vi "CR-导丝划痕检测1.vi"(8 "error in (no error)":errorcluster caption="错误输入（无错误）", 11 "名称或相对路径":string="Template Program") -> (0 "error in (no error) 2":errorcluster caption="错误输入（无错误）")   [LabVIEW 2017]
uses:
  Picture/SaveButtom.ctl
  Global System.vi
  <vilib>/Utility/xml.llb/Write to XML File(string).vi
panel:
  in  "获取图像":bool
  in  "ROI获取":bool
  in  "创建模板":bool
  in  "保存图像":bool
  out "添加的路径":path
  in  "刷新":bool
  in  "测试按钮":bool
  in  "保存按钮":bool
  in  "Main":enum32{"主参数", "模板匹配参数 ", "测试效果"}(tab)
  in  "导丝划痕检测1基础参数":T1={"IsNorImage"=TRUE, "Exposure Values"=100289, "ImagePath"=path "C:/Users/hedongpo/Desktop/514-hdp/Alignment Assemble System/Test Picture/B/3.bmp"} caption="参数界面" {"Exposure Values" scale=0.0..200000.0}
  in  "导丝划痕检测1参数":T3={"Rectangle"={"Left"=0, "Top"=0, "Right"=0, "Bottom"=0, "Rotation"=0.0}, "Algorithm "=2, "Parameters"={"Number of Matches Requested"=1, "Minimum Match Score"=800.0, "Angle Ranges"=[{"Start Angle"=-180.0, "End Angle"=180.0}]}, "Advanced Options "=[{"Item"=102, "Value"=10.0}, {"Item"=106, "Value"=300.0}, {"Item"=107, "Value"=0.0}, {"Item"=108, "Value"=6.0}, {"Item"=109, "Value"=1.0}, {"Item"=114, "Value"=25.0}, {"Item"=111, "Value"=20.0}, {"Item"=112, "Value"=10.0}, {"Item"=113, "Value"=20.0}, {"Item"=103, "Value"=1.0}, {"Item"=104, "Value"=20.0}, {"Item"=105, "Value"=0.0}, {"Item"=100, "Value"=5.0}], "模板路径"=path "", "Color Plane "=0} {"Color Plane" items=["Red", "Green", "Blue", "Hue", "Saturation", "Luminance", "Value", "Intensity"]; "Advanced Options"."Item" items=["LD Sampling - Minimum Constrast"=0, "LD Sampling - Enable Subpixel Accuracy"=1, "LD Sampling - Search Strategy"=2, "LD Sampling - Subpixel Iterations"=3, "LD Sampling - Subpixel Tolerance"=4, "LD Sampling - Initial Match List Length"=5, "LD Sampling - Match List Reduction Factor"=6, "LD Sampling - Initial Step Size"=7, "LD Sampling - Intermediate Angular Accuracy"=8, "-"=9, "Pyramid - Max Pyramid Level"=100, "Pyramid - Minimum Contrast"=102, "Pyramid - Enable Subpixel Accuracy"=103, "Pyramid - Subpixel Iterations"=104, "Pyramid - Subpixel Tolerance"=105, "Pyramid - Initial Match List Length"=106, "Pyramid - Match List Reduction Factor"=107, "Pyramid - Intermediate Angular Accuracy"=108, "Pyramid - Process Border Matches"=109, "Pyramid - Min Match Separation Distance"=111, "Pyramid - Min Match Separation Angle"=112, "Pyramid - Max Match Overlap"=113, "Pyramid - Max Cache in MB"=114, "Pyramid - Clear Cache"=115, "-"=116, "Enable Defect Map"=200]; "Algorithm" items=["All", "Low Discrepancy Sampling", "Grayscale Value Pyramid", "Gradients Pyramid"]; "Rectangle"."Rotation" format="%.2f"; "Rectangle"."Left" scale=0.0..1024.0; "Rectangle"."Right" scale=0.0..1024.0}
  out "结果":bool
  out "原始图像":T4(plugin-control)
  out "路径输出":path
  in  "Vision Paramter Save Buttom":T5
  out "system time":string
  in  "取消按钮":bool
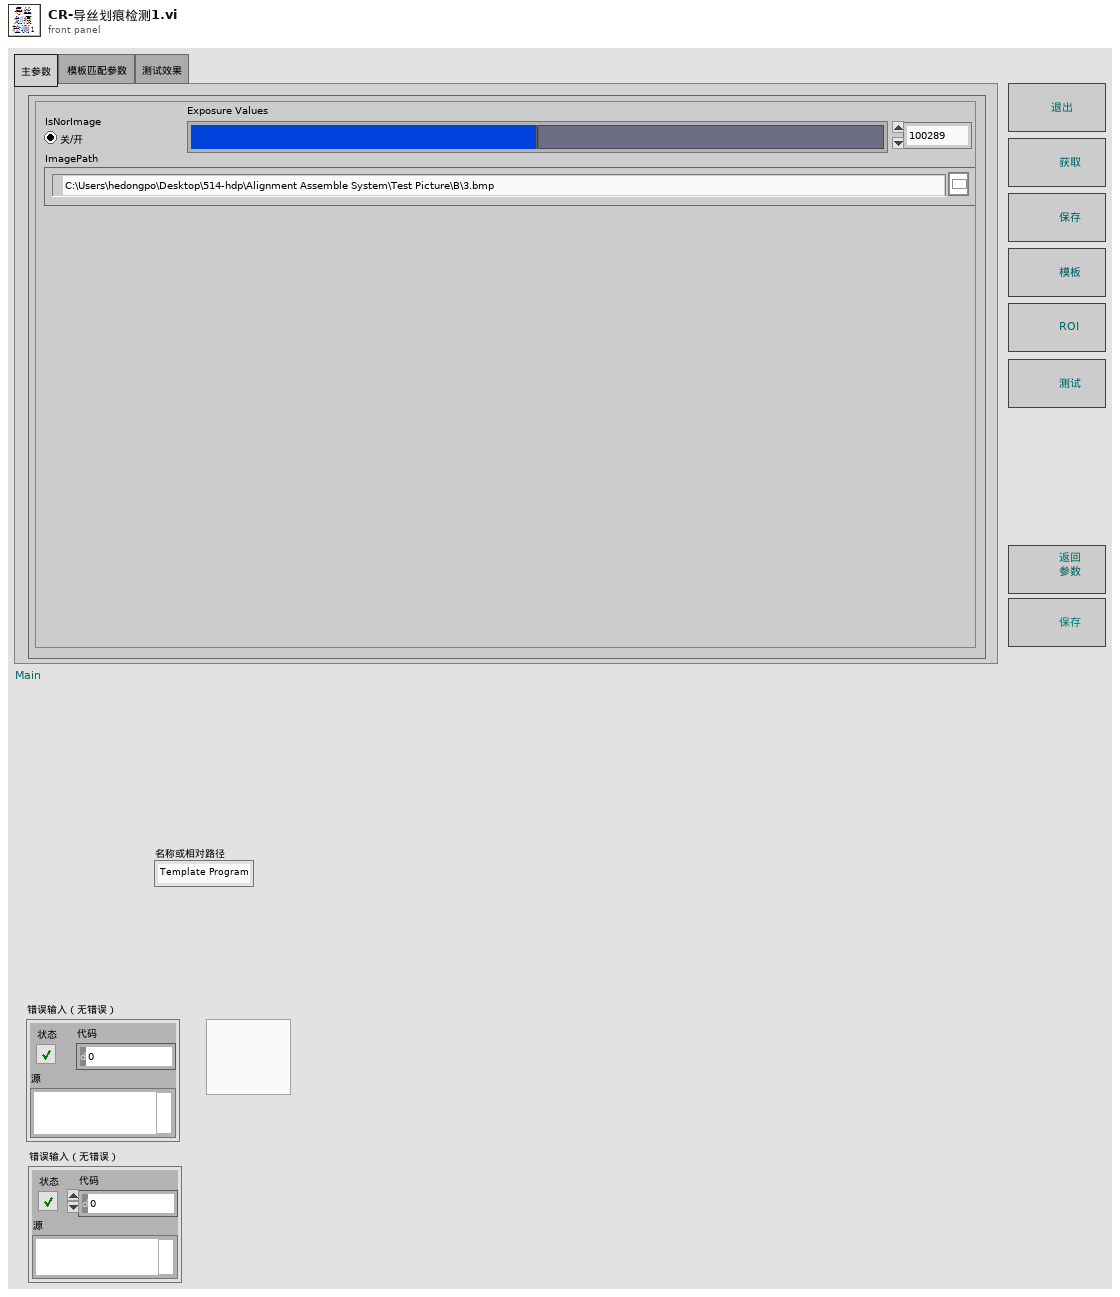
[diagram p1: front panel]
types:
  T1 = cluster{"IsNorImage":bool, "Exposure Values":u32, "ImagePath":path}
  T2 = typedef "IMAQ Rectangle" = cluster{"Left":i32, "Top":i32, "Right":i32, "Bottom":i32, "Rotation":dbl}
  T3 = cluster{"Rectangle":T2, "Algorithm ":i32, "Parameters":cluster{"Number of Matches Requested":i32, "Minimum Match Score":sgl, "Angle Ranges":cluster{"Start Angle":sgl, "End Angle":sgl}[]}, "Advanced Options ":cluster{"Item":u16, "Value":dbl}[], "模板路径":path, "Color Plane ":i32}
  T4 = typedef "IMAQ Image.ctl" = refnum<image>
  T5 = typedef "SaveButtom.ctl" = bool
  T6 = cluster{"index":i32, "this vi":refnum<vi>, "error out":errorcluster}
  T7 = cluster{"master data":string, "priority":u16, "secondary data":string[]}
  T8 = cluster{"case name":string[], "queue array":refnum<queue>[]}
  T9 = cluster{"Global Rectangle":i32[], "Contours":cluster{"Contour Type":u32, "ROI Type":u32, "Points":i32[]}[]}
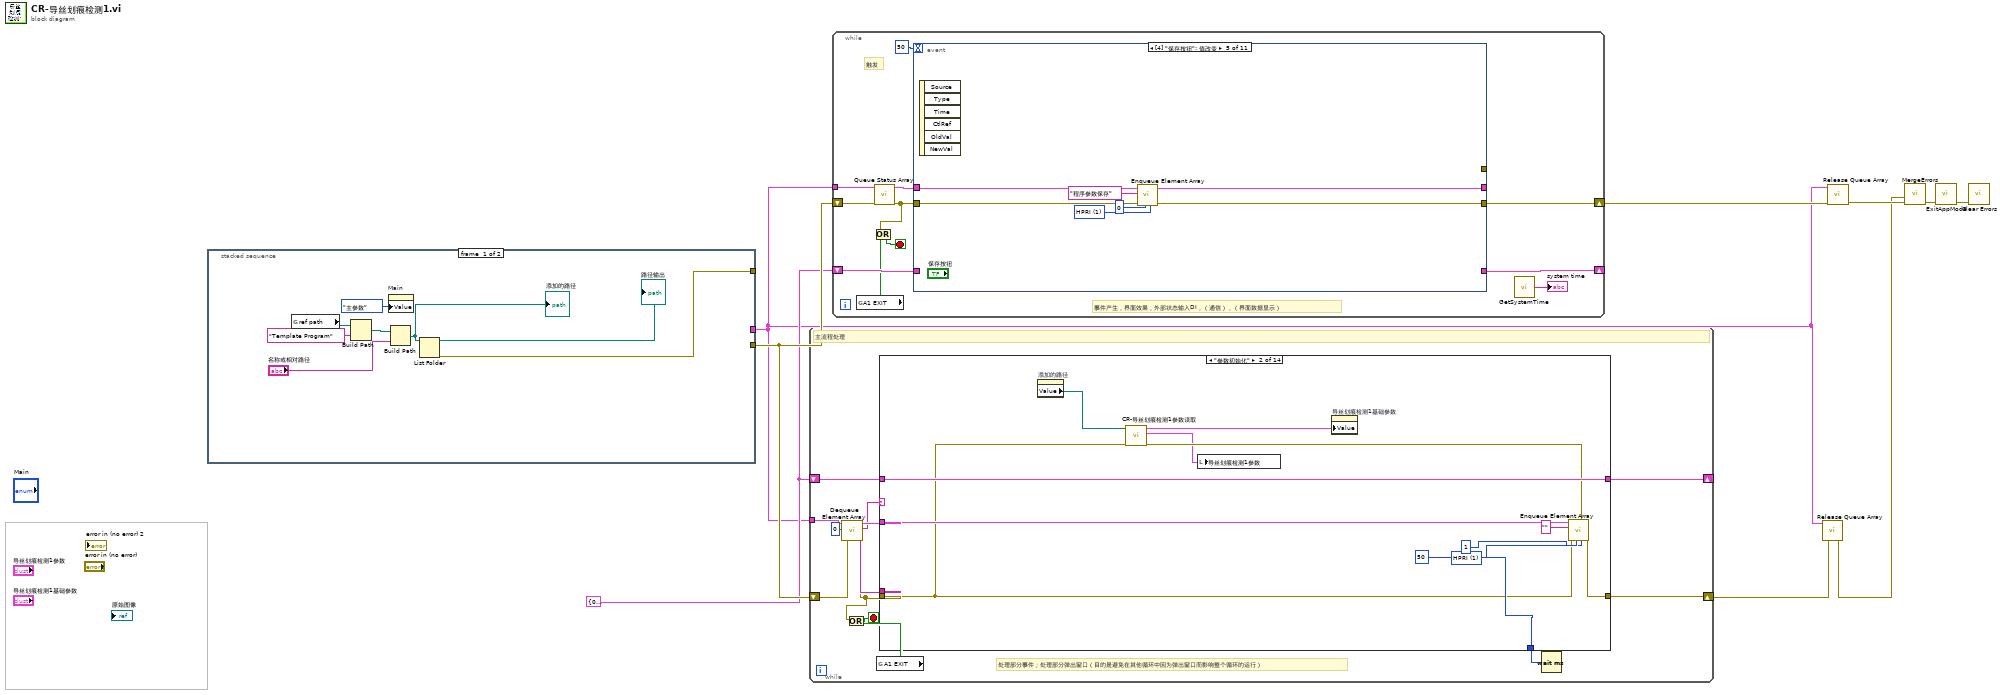
[diagram p0: block diagram]
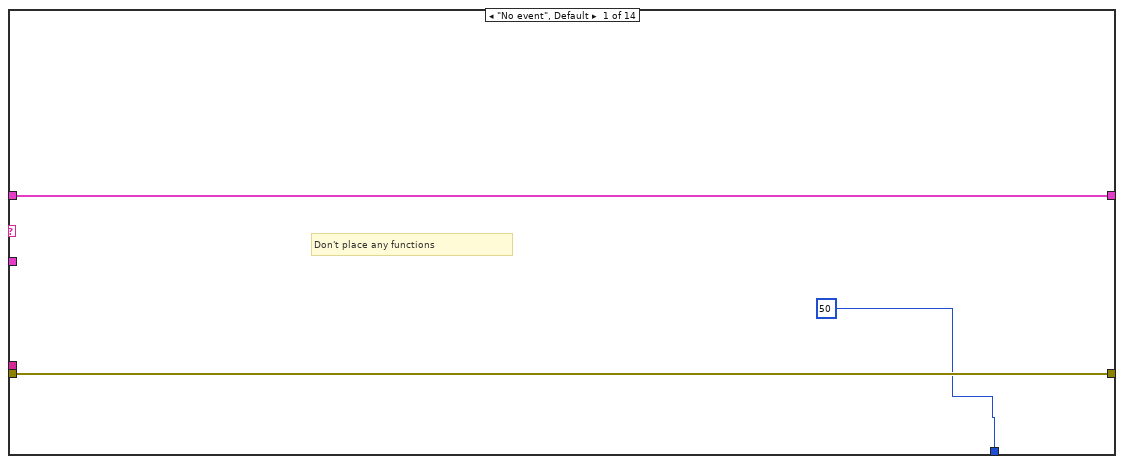
[diagram p2: hidden frame]
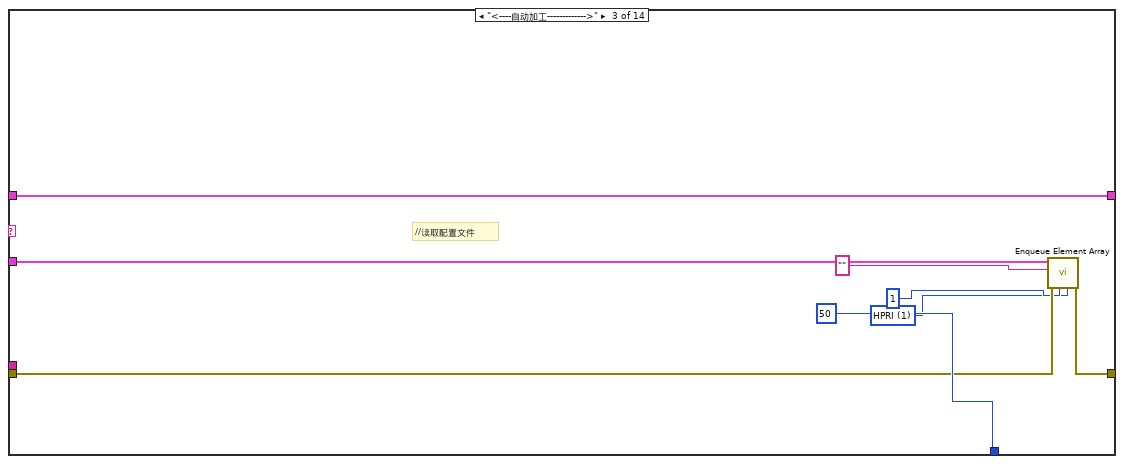
[diagram p3: hidden frame]
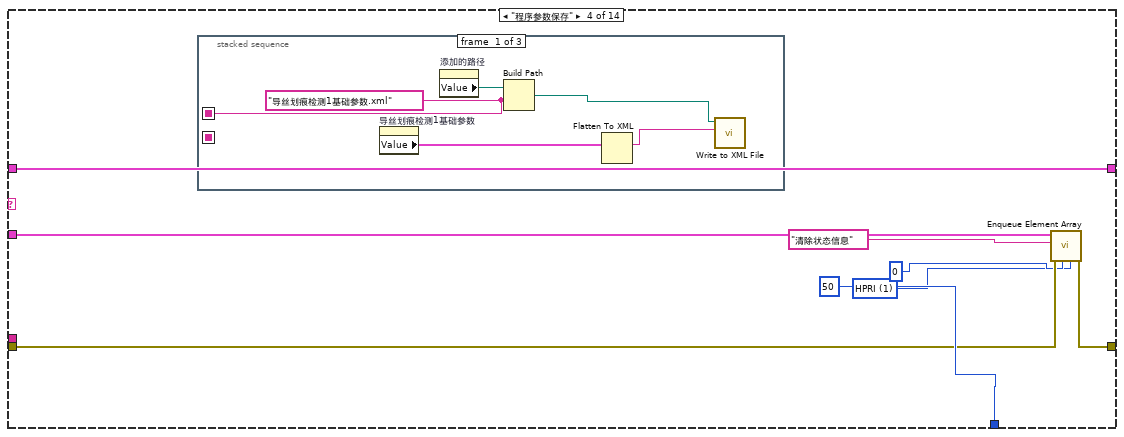
[diagram p4: hidden frame]
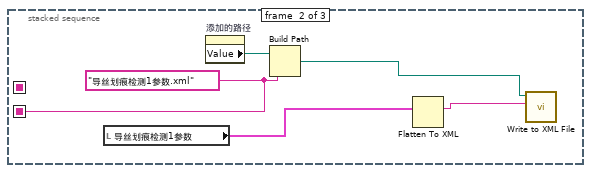
[diagram p5: hidden frame]
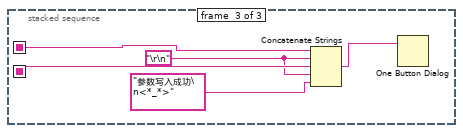
[diagram p6: hidden frame]
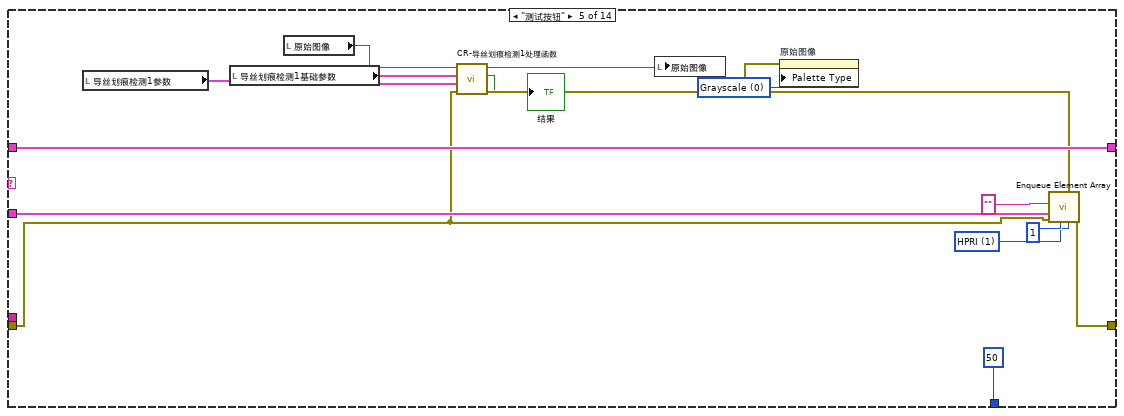
[diagram p7: hidden frame]
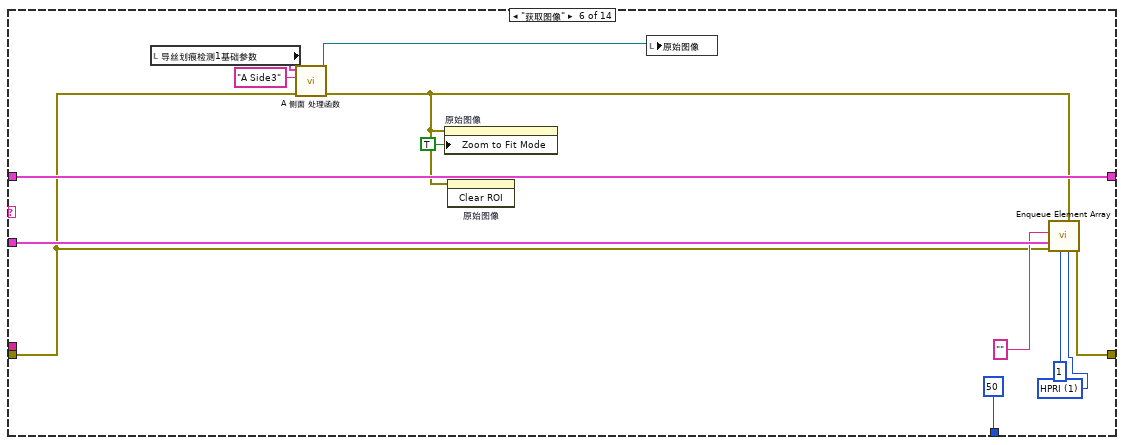
[diagram p8: hidden frame]
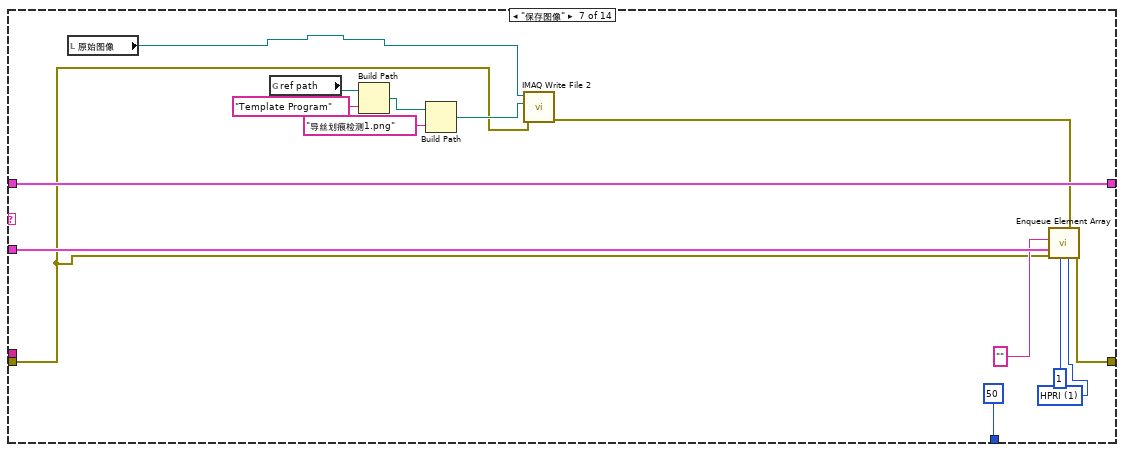
[diagram p9: hidden frame]
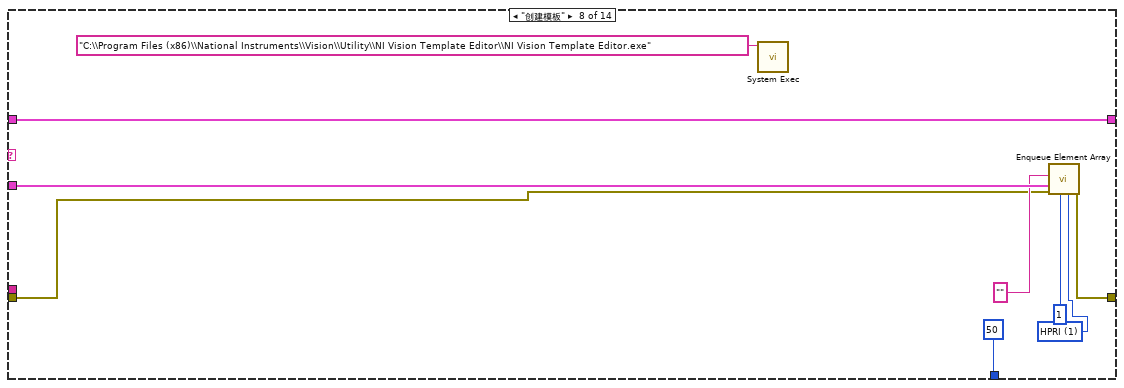
[diagram p10: hidden frame]
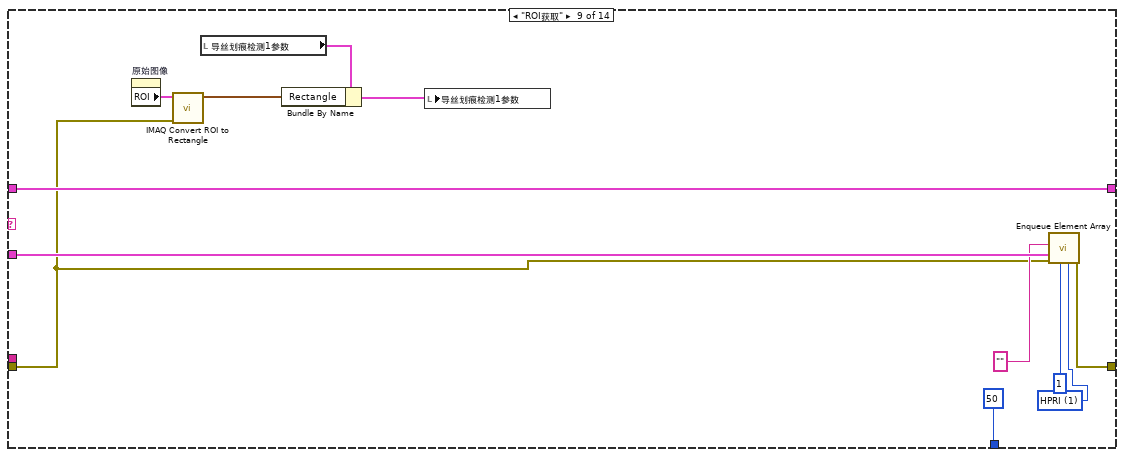
[diagram p11: hidden frame]
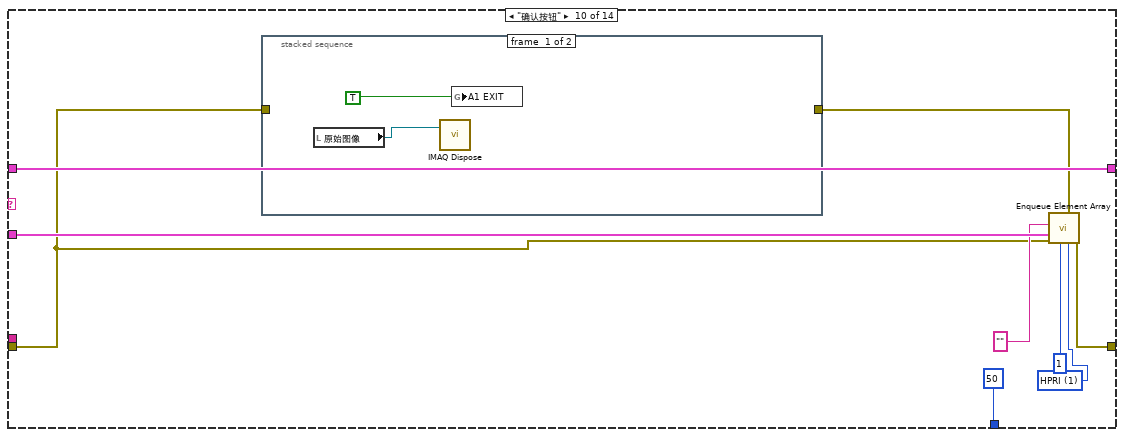
[diagram p12: hidden frame]
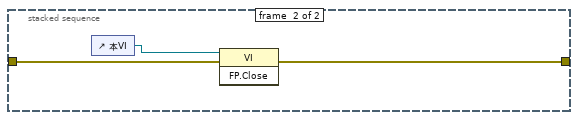
[diagram p13: hidden frame]
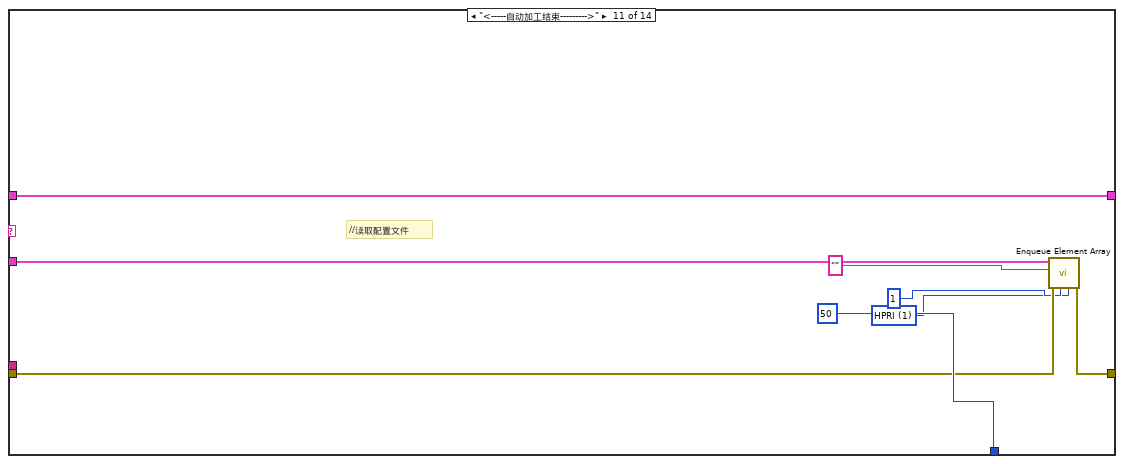
[diagram p14: hidden frame]
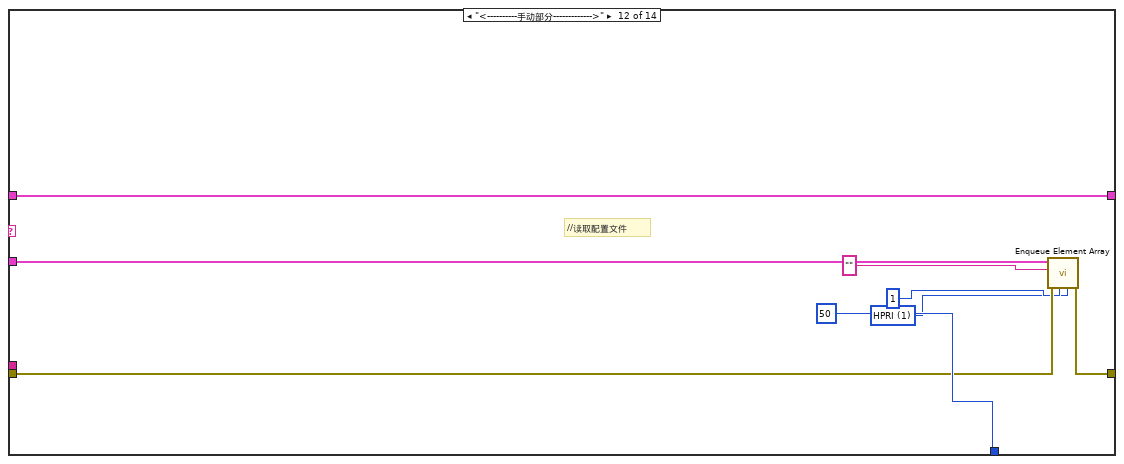
[diagram p15: hidden frame]
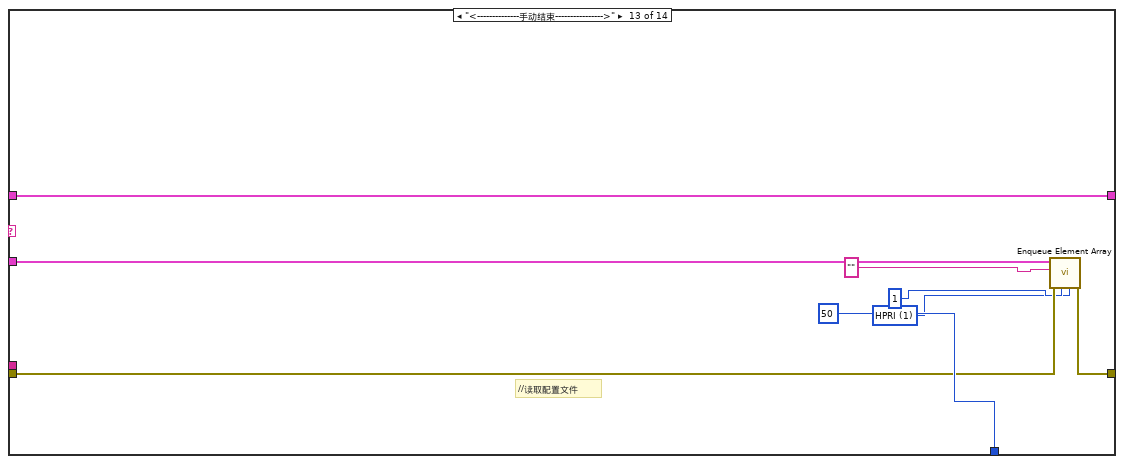
[diagram p16: hidden frame]
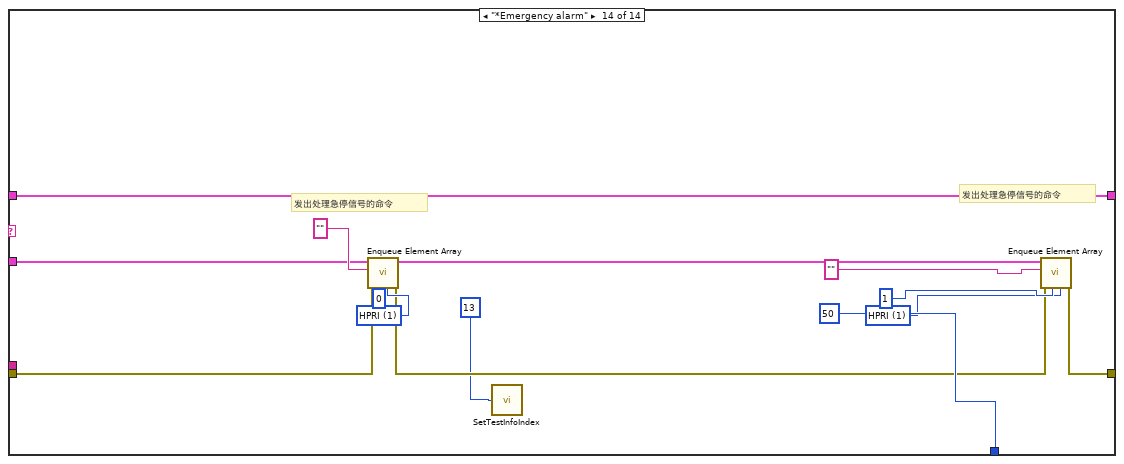
[diagram p17: hidden frame]
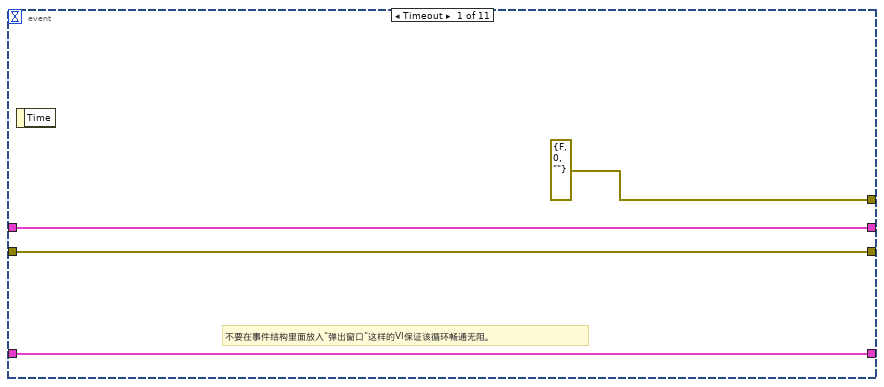
[diagram p18: hidden frame]
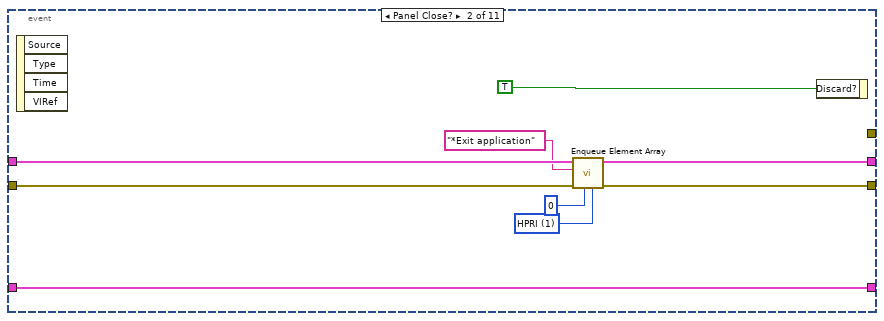
[diagram p19: hidden frame]
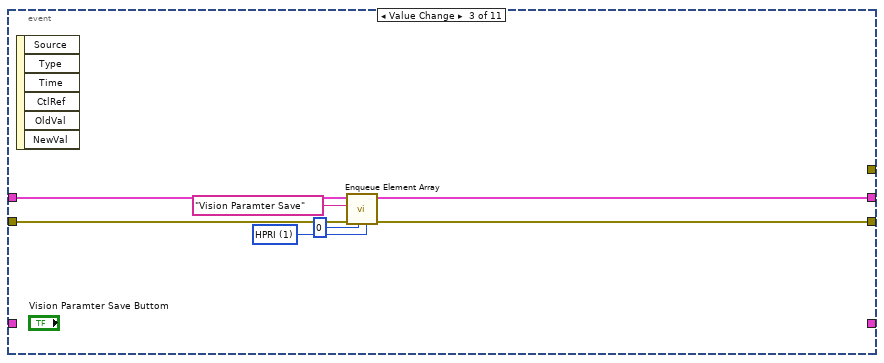
[diagram p20: hidden frame]
diagram:
  w4 = T6 {"index"=0, "this vi"=refnum, "error out"={"status"=FALSE, "code"=0, "source"=""}} ("parameter buffer")
  n1 = stacked-sequence {
    tunnel: [w15 _] -> _
    tunnel: [_ w19] -> w5
    tunnel: [_ w18] -> w1
    frame #0 {
      n2 = global read "Global System.vi" "ref path"() -> (w13:path)
      n3 = Build Path(base path=w13, name or relative path="Template Program" ("名称或相对路径")) -> (appended path=w11:path)
      n4 = property on="Main" class="TabCtl (严格)"("Value"=enum32{"主参数", "模板匹配参数 ", "测试效果"}."主参数" ("Main")) -> ()  [unwired: 2 in, 2 out]
      n5 = Build Path(base path=w11, name or relative path="名称或相对路径") -> (appended path=w17:path)
      "添加的路径" <- w17
      n6 = List Folder(path=w17) -> (path out=→"路径输出":path, error out=w15:errorcluster)  [unwired: 3 in, 2 out]
    }
    frame #1 {
      w27 = string[] ["comm queue1", "data queue 11", "data queue 12", "data queue 13", "data queue 14"]  # queue name
      w28 = 4  # queue num
      w29 = T7 {"master data"="", "priority"=0, "secondary data"=[]}  # element data type
      n7 = call "Obtain Queue Array.vi"("queue name"=w27, "element data type"=w29, "queue num"=w28) -> ("error out"=w23:errorcluster, "queue out"=w24:T8)  [unwired: 2 in, 1 out]
      n8 = call "Enqueue Element Array.vi"("queue index"=0, "error in"=w23, "master data"="参数初始化", "queue in"=w24) -> ("error out"=w22:errorcluster, "queue out"=w21:T8)  [unwired: 6 in]
      n9 = disable-structure shown="启用" {
        disable-tunnel: w22 -> [w35 w36]
        disable-tunnel: w21 -> [w34 w37]
        disable-tunnel: "Loading Variable" ("master data") -> [w33 _]
        disable-tunnel: [w31 w36] -> w19
        disable-tunnel: [w30 w37] -> w18
        frame Disabled {
          n10 = call "Enqueue Element Array.vi"("queue index"=12, "error in"=w35, "master data"=w33, "queue in"=w34) -> ("error out"=w31:errorcluster, "queue out"=w30:T8)  [unwired: 6 in]
        }
        frame Enabled {
        }
      }
    }
  }
  n11 = while {
    shift-right: [w50] -> w3
    shift-left: w5 -> [w41]
    shift-right: [w47] -> _
    shift-left: w4 -> [w48]
    tunnel: w1 -> [w43]
    stop <- w38 stop-if-true
    # "处理部分事件；处理部分弹出窗口（目的是避免在其他循环中因为弹出窗口而影响整个循环的运行）"
    # "主流程处理"
    n12 = call "Dequeue Element Array.vi"("queue in"=w43, "queue index"=0, "error in"=w41) -> ("queue out"=w46:T8, "master data"=w45:string, "secondary data"=w44:string[], "error out"=w40:errorcluster)  [unwired: 2 in, 1 out]
    n13 = global read "Global System.vi" "A1 EXIT"() -> (w39:bool)
    n14 = Or(x=w40, y=w39) -> (x .or. y?=w38:bool)
    n15 = case shown="\"参数初始化\"" w45 {
      tunnel: w46 -> [_ w64 w72 w74 w110 w123 w138 w147 w159 w168 w181 w189 w197 w203]
      tunnel: w40 -> [w52 w57 w68 w78 w103 w114 w125 w141 w152 w162 w177 w185 w193 w200]
      tunnel: [w52 w63 w71 w80 w109 w122 w137 w146 w158 w167 w180 w188 w196 w211] -> w50
      tunnel: [50 50 50 50 50 50 50 50 50 50 50 50 50 50] -> w49
      tunnel: w48 -> [w53 w59 w69 w75 w105 w118 w133 w142 w154 w163 w178 w186 w194 w209]
      tunnel: [w53 w59 w69 w75 w105 w118 w133 w142 w154 w163 w178 w186 w194 w209] -> w47
      tunnel: w44 -> [_ _ _ _ _ _ _ _ _ _ _ _ _ _]
      frame "No event", Default {
        # "Don't place any functions"
      }
      frame "参数初始化" {
        w60 = u16 1 items=["HPRI"=1, "LPRI"=0] ("priority")
        n16 = property on="添加的路径" class="Path"() -> ("Value"=w58:path)  [unwired: 2 in, 2 out]
        n17 = call "CR-导丝划痕检测1参数读取.vi"("error in (no error)"=w57, "基路径"=w58) -> ("error out"=w56:errorcluster, "导丝划痕检测1参数"=w54:T3, "导丝划痕检测1基础参数"=w55:T1)  [unwired: 6 in]
        n18 = local write "导丝划痕检测1参数"(w54) -> ()
        n19 = property on="导丝划痕检测1基础参数" class="Clust (严格)"("Value"=w55) -> ()  [unwired: 2 in, 2 out]
        n20 = call "Enqueue Element Array.vi"("priority"=w60, "device error in"=w56, "queue index"=1, "error in"=w57, "master data"="" ("Element 1"), "queue in"=w64) -> ("error out"=w63:errorcluster)  [unwired: 4 in, 1 out]
      }
      frame "<----自动加工------------->" {
        w66 = u16 1 items=["HPRI"=1, "LPRI"=0] ("priority")
        # "//读取配置文件"
        n21 = call "Enqueue Element Array.vi"("priority"=w66, "queue index"=1, "error in"=w68, "master data"="" ("Element 1"), "queue in"=w72) -> ("error out"=w71:errorcluster)  [unwired: 5 in, 1 out]
      }
      frame "程序参数保存" {
        w76 = u16 1 items=["HPRI"=1, "LPRI"=0] ("priority")
        n22 = stacked-sequence {
          seq-local: [w82 _ _] -> [_ _ w95]
          seq-local: [_ w88 _] -> [_ _ w93]
          frame #0 {
            w82 = "导丝划痕检测1基础参数.xml" ("名称或相对路径")
            n23 = property on="导丝划痕检测1基础参数" class="Clust (严格)"() -> ("Value"=w85:T1)  [unwired: 2 in, 2 out]
            n24 = property on="添加的路径" class="Path"() -> ("Value"=w86:path)  [unwired: 2 in, 2 out]
            n25 = Build Path(base path=w86, name or relative path=w82) -> (appended path=w83:path)
            n26 = Flatten To XML(anything=w85) -> (xml string=w84:string)
            n27 = call-poly <vilib>:"Write to XML File.vi"("XML Input"=w84, "XML File Path"=w83) -> ()  [unwired: 7 in, 3 out]
          }
          frame #1 {
            w88 = "导丝划痕检测1参数.xml" ("名称或相对路径")
            n28 = local read "导丝划痕检测1参数"() -> (w87:T3)
            n29 = property on="添加的路径" class="Path"() -> ("Value"=w91:path)  [unwired: 2 in, 2 out]
            n30 = Build Path(base path=w91, name or relative path=w88) -> (appended path=w89:path)
            n31 = Flatten To XML(anything=w87) -> (xml string=w90:string)
            n32 = call-poly <vilib>:"Write to XML File.vi"("XML Input"=w90, "XML File Path"=w89) -> ()  [unwired: 7 in, 3 out]
          }
          frame #2 {
            w92 = "\r\n"
            n33 = Concatenate Strings(w95, w92, w93, w92, "参数写入成功\n<*_*>" ("消息")) -> (w94:string)
            n34 = One Button Dialog(message=w94) -> ()  [unwired: 1 in, 1 out]
          }
        }
        n35 = call "Enqueue Element Array.vi"("priority"=w76, "queue index"=0, "error in"=w78, "master data"="清除状态信息" ("Element 1"), "queue in"=w74) -> ("error out"=w80:errorcluster)  [unwired: 5 in, 1 out]
      }
      frame "测试按钮" {
        w98 = u32 0 items=["Grayscale", "Binary", "Gradient", "Rainbow", "Temperature", "User Defined", "Binary 16 Bit", "Gradient 16 Bit", "Rainbow 16 Bit", "Temperature 16 Bit", "User Defined 16 Bit"] ("Palette:Palette Type")
        w106 = u16 1 items=["HPRI"=1, "LPRI"=0] ("priority")
        n36 = local read "导丝划痕检测1参数"() -> (w101:T3)
        n37 = local read "导丝划痕检测1基础参数"() -> (w104:T1)
        n38 = local read "原始图像"() -> (w100:T4)
        n39 = call "CR-导丝划痕检测1处理函数.vi"("error in (no error)"=w103, "UI电源线正面标签1参数"=w101, "电源线正面标签1基础参数"=w104, "Image in"=w100) -> ("error out"=w99:errorcluster, "j结果"=→"结果":bool, "Image out"=w102:T4)  [unwired: 4 in, 1 out]
        n40 = local write "原始图像"(w102) -> ()
        n41 = property on="原始图像" class="ImageControl"(error in=w99, "Palette Type"=w98) -> ()  [unwired: 1 in, 2 out]
        n42 = call "Enqueue Element Array.vi"("priority"=w106, "device error in"=w99, "queue index"=1, "error in"=w103, "master data"="" ("Element 1"), "queue in"=w110) -> ("error out"=w109:errorcluster)  [unwired: 4 in, 1 out]
      }
      frame "获取图像" {
        w119 = u16 1 items=["HPRI"=1, "LPRI"=0] ("priority")
        n43 = local read "导丝划痕检测1基础参数"() -> (w116:T1)
        n44 = call "A 侧面 处理函数.vi"("error in (no error)"=w114, "Image Name"="A Side3", "ParamsUI"=w116) -> ("error out"=w112:errorcluster, "Image out"=w115:T4)  [unwired: 5 in, 2 out]
        n45 = property on="原始图像" class="ImageControl"(error in=w112, "Zoom to Fit Mode"=TRUE) -> ()  [unwired: 1 in, 2 out]
        n46 = invoke on="原始图像" class="ImageControl" method="Clear ROI"(error in=w112) -> ()  [unwired: 2 in, 3 out]
        n47 = local write "原始图像"(w115) -> ()
        n48 = call "Enqueue Element Array.vi"("priority"=w119, "device error in"=w112, "queue index"=1, "error in"=w114, "master data"="" ("Element 1"), "queue in"=w123) -> ("error out"=w122:errorcluster)  [unwired: 4 in, 1 out]
      }
      frame "保存图像" {
        w134 = u16 1 items=["HPRI"=1, "LPRI"=0] ("priority")
        n49 = local read "原始图像"() -> (w126:T4)
        n50 = global read "Global System.vi" "ref path"() -> (w132:path)
        n51 = Build Path(base path=w132, name or relative path="Template Program" ("名称或相对路径")) -> (appended path=w130:path)
        n52 = Build Path(base path=w130, name or relative path="导丝划痕检测1.png" ("名称或相对路径")) -> (appended path=w128:path)
        n53 = call-poly "IMAQ Write File 2"("error in (no error)"=w125, "File Path"=w128, "Image"=w126) -> ("error out"=w127:errorcluster)  [unwired: 7 in, 1 out]
        n54 = call "Enqueue Element Array.vi"("priority"=w134, "device error in"=w127, "queue index"=1, "error in"=w125, "master data"="" ("Element 1"), "queue in"=w138) -> ("error out"=w137:errorcluster)  [unwired: 4 in, 1 out]
      }
      frame "创建模板" {
        w143 = u16 1 items=["HPRI"=1, "LPRI"=0] ("priority")
        n55 = call <vilib>:"System Exec.vi"("command line"="C:\\Program Files (x86)\\National Instruments\\Vision\\Utility\\NI Vision Template Editor\\NI Vision Template Editor.exe") -> ()  [unwired: 7 in, 4 out]
        n56 = call "Enqueue Element Array.vi"("priority"=w143, "queue index"=1, "error in"=w141, "master data"="" ("Element 1"), "queue in"=w147) -> ("error out"=w146:errorcluster)  [unwired: 5 in, 1 out]
      }
      frame "ROI获取" {
        w155 = u16 1 items=["HPRI"=1, "LPRI"=0] ("priority")
        n57 = property on="原始图像" class="ImageControl"() -> ("ROI"=w153:T9)  [unwired: 2 in, 2 out]
        n58 = call "IMAQ Convert ROI to Rectangle"("error in (no error)"=w152, "ROI Descriptor"=w153) -> ("Rectangle"=w150:T2)  [unwired: 7 in, 1 out]
        n59 = local read "导丝划痕检测1参数"() -> (w151:T3)
        n60 = Bundle By Name(cluster=w151, "Rectangle"=w150) -> (w149:T3)
        n61 = local write "导丝划痕检测1参数"(w149) -> ()
        n62 = call "Enqueue Element Array.vi"("priority"=w155, "queue index"=1, "error in"=w152, "master data"="" ("Element 1"), "queue in"=w159) -> ("error out"=w158:errorcluster)  [unwired: 5 in, 1 out]
      }
      frame "确认按钮" {
        w164 = u16 1 items=["HPRI"=1, "LPRI"=0] ("priority")
        n63 = stacked-sequence {
          tunnel: w162 -> [_ w173]
          tunnel: [_ w172] -> w161
          frame #0 {
            n64 = local read "原始图像"() -> (w170:T4)
            n65 = call "IMAQ Dispose"("Image"=w170) -> ()  [unwired: 5 in, 1 out]
            n66 = global write "Global System.vi" "A1 EXIT"(TRUE ("EXIT")) -> ()
          }
          frame #1 {
            n67 = control-ref of="本VI"() -> (w174:refnum<vi>)
            n68 = invoke class="VI" method="FP.Close"(reference=w174, error in=w173) -> (error out=w172:errorcluster)  [unwired: 1 in, 2 out]
          }
        }
        n69 = call "Enqueue Element Array.vi"("priority"=w164, "device error in"=w161, "queue index"=1, "error in"=w162, "master data"="" ("Element 1"), "queue in"=w168) -> ("error out"=w167:errorcluster)  [unwired: 4 in, 1 out]
      }
      frame "<-----自动加工结束--------->" {
        w175 = u16 1 items=["HPRI"=1, "LPRI"=0] ("priority")
        # "//读取配置文件"
        n70 = call "Enqueue Element Array.vi"("priority"=w175, "queue index"=1, "error in"=w177, "master data"="" ("Element 1"), "queue in"=w181) -> ("error out"=w180:errorcluster)  [unwired: 5 in, 1 out]
      }
      frame "<----------手动部分------------->" {
        w183 = u16 1 items=["HPRI"=1, "LPRI"=0] ("priority")
        # "//读取配置文件"
        n71 = call "Enqueue Element Array.vi"("priority"=w183, "queue index"=1, "error in"=w185, "master data"="" ("Element 1"), "queue in"=w189) -> ("error out"=w188:errorcluster)  [unwired: 5 in, 1 out]
      }
      frame "<--------------手动结束---------------->" {
        w191 = u16 1 items=["HPRI"=1, "LPRI"=0] ("priority")
        # "//读取配置文件"
        n72 = call "Enqueue Element Array.vi"("priority"=w191, "queue index"=1, "error in"=w193, "master data"="" ("Element 1"), "queue in"=w197) -> ("error out"=w196:errorcluster)  [unwired: 5 in, 1 out]
      }
      frame "*Emergency alarm" {
        w206 = u16 1 items=["HPRI"=1, "LPRI"=0] ("priority")
        w207 = u16 1 items=["HPRI"=1, "LPRI"=0] ("priority")
        # "发出处理急停信号的命令"
        # "发出处理急停信号的命令"
        n73 = call "Enqueue Element Array.vi"("priority"=w206, "queue index"=0, "error in"=w200, "master data"="" ("Element 1"), "queue in"=w203) -> ("error out"=w201:errorcluster, "queue out"=w202:T8)  [unwired: 5 in]
        n74 = call "SetTestInfoIndex.vi"("test info index"=13) -> ()
        n75 = call "Enqueue Element Array.vi"("priority"=w207, "queue index"=1, "error in"=w201, "master data"="" ("Element 1"), "queue in"=w202) -> ("error out"=w211:errorcluster)  [unwired: 5 in, 1 out]
      }
    }
    n76 = Wait (ms)(milliseconds to wait=w49) -> ()  [unwired: 1 out]
  }
  n77 = while {
    shift-right: [w216] -> w6
    shift-left: w5 -> [w220]
    shift-right: [w218] -> _
    shift-left: w4 -> [w219]
    tunnel: w1 -> [w222]
    stop <- w213 stop-if-true
    # "触发"
    # "事件产生，界面效果，外部状态输入DI，（通信），（界面数据显示）"
    n78 = global read "Global System.vi" "A1 EXIT"() -> (w214:bool)
    n79 = call "Queue Status Array.vi"("error in (no error)"=w220, "queue in"=w222) -> ("error out"=w215:errorcluster, "queue out"=w217:T8)  [unwired: 4 in]
    n80 = Or(x=w215, y=w214) -> (x .or. y?=w213:bool)
    n81 = event shown="[4] \"保存按钮\": 值改变" {
      selector: _ -> [_ _ _ _ _ _ _ _ _ _ _]
      dyn-events: _ -> [_ _ _ _ _ _ _ _ _ _ _]
      timeout: 50 -> [_ _ _ _ _ _ _ _ _ _ _]
      tunnel: w219 -> [w227 w235 _ _ _ _ _ _ _ _ _]
      tunnel: [w227 w235 _ _ _ _ _ _ _ _ _] -> w218
      tunnel: [errorcluster {"status"=FALSE, "code"=0, "source"=""} ("error out") _ _ _ _ _ _ _ _ _ _] -> _
      tunnel: w217 -> [w225 w234 w240 w247 w254 w262 w269 w276 w284 w292 w300]
      tunnel: w215 -> [w224 w233 w239 w246 w253 w261 w268 w275 w283 w291 w299]
      tunnel: [w224 w232 w237 w244 w251 w259 w266 w273 w281 w289 w297] -> w216
      tunnel: [w225 w231 w238 w245 w252 w260 w267 w274 w282 w290 w298] -> _
      event Timeout {
        # "不要在事件结构里面放入\"弹出窗口\"这样的VI保证该循环畅通无阻。"
        n82 = event-data() -> ()  [unwired: 1 in, 1 out]
      }
      event Panel Close? {
        w229 = u16 1 items=["HPRI"=1, "LPRI"=0] ("priority")
        n83 = event-data() -> ()  [unwired: 1 in, 4 out]
        n84 = call "Enqueue Element Array.vi"("priority"=w229, "queue index"=0, "error in"=w233, "master data"="*Exit application", "queue in"=w234) -> ("error out"=w232:errorcluster, "queue out"=w231:T8)  [unwired: 5 in]
        n85 = event-data("Discard?"=TRUE) -> ()  [unwired: 1 in, 1 out]
      }
      event Value Change {
        w242 = u16 1 items=["HPRI"=1, "LPRI"=0] ("priority")
        n86 = event-data() -> ()  [unwired: 1 in, 6 out]
        n87 = call "Enqueue Element Array.vi"("priority"=w242, "queue index"=0, "error in"=w239, "master data"="Vision Paramter Save", "queue in"=w240) -> ("error out"=w237:errorcluster, "queue out"=w238:T8)  [unwired: 5 in]
      }
      event "取消按钮": Value Change {
        w249 = u16 1 items=["HPRI"=1, "LPRI"=0] ("priority")
        n88 = event-data() -> ()  [unwired: 1 in, 6 out]
        n89 = call "Enqueue Element Array.vi"("priority"=w249, "queue index"=0, "error in"=w246, "master data"="确认按钮", "queue in"=w247) -> ("error out"=w244:errorcluster, "queue out"=w245:T8)  [unwired: 5 in]
      }
      event "保存按钮": Value Change {
        w256 = u16 1 items=["HPRI"=1, "LPRI"=0] ("priority")
        n90 = event-data() -> ()  [unwired: 1 in, 6 out]
        n91 = call "Enqueue Element Array.vi"("priority"=w256, "queue index"=0, "error in"=w253, "master data"="程序参数保存", "queue in"=w254) -> ("error out"=w251:errorcluster, "queue out"=w252:T8)  [unwired: 5 in]
      }
      event "获取图像": Value Change {
        w264 = u16 1 items=["HPRI"=1, "LPRI"=0] ("priority")
        n92 = event-data() -> ()  [unwired: 1 in, 6 out]
        n93 = property on="Main" class="TabCtl (严格)"("Value"=enum32{"主参数", "模板匹配参数 ", "测试效果"}."测试效果" ("Main")) -> ()  [unwired: 2 in, 2 out]
        n94 = call "Enqueue Element Array.vi"("priority"=w264, "queue index"=0, "error in"=w261, "master data"="获取图像", "queue in"=w262) -> ("error out"=w259:errorcluster, "queue out"=w260:T8)  [unwired: 5 in]
      }
      event "保存图像": Value Change {
        w271 = u16 1 items=["HPRI"=1, "LPRI"=0] ("priority")
        n95 = event-data() -> ()  [unwired: 1 in, 6 out]
        n96 = call "Enqueue Element Array.vi"("priority"=w271, "queue index"=0, "error in"=w268, "master data"="保存图像", "queue in"=w269) -> ("error out"=w266:errorcluster, "queue out"=w267:T8)  [unwired: 5 in]
      }
      event "创建模板": Value Change {
        w278 = u16 1 items=["HPRI"=1, "LPRI"=0] ("priority")
        n97 = event-data() -> ()  [unwired: 1 in, 6 out]
        n98 = call "Enqueue Element Array.vi"("priority"=w278, "queue index"=0, "error in"=w275, "master data"="创建模板", "queue in"=w276) -> ("error out"=w273:errorcluster, "queue out"=w274:T8)  [unwired: 5 in]
      }
      event "ROI获取": Value Change {
        w286 = u16 1 items=["HPRI"=1, "LPRI"=0] ("priority")
        n99 = event-data() -> ()  [unwired: 1 in, 6 out]
        n100 = property on="Main" class="TabCtl (严格)"("Value"=enum32{"主参数", "模板匹配参数 ", "测试效果"}."模板匹配参数 " ("Main")) -> ()  [unwired: 2 in, 2 out]
        n101 = call "Enqueue Element Array.vi"("priority"=w286, "queue index"=0, "error in"=w283, "master data"="ROI获取", "queue in"=w284) -> ("error out"=w281:errorcluster, "queue out"=w282:T8)  [unwired: 5 in]
      }
      event "测试按钮": Value Change {
        w294 = u16 1 items=["HPRI"=1, "LPRI"=0] ("priority")
        n102 = event-data() -> ()  [unwired: 1 in, 6 out]
        n103 = property on="Main" class="TabCtl (严格)"("Value"=enum32{"主参数", "模板匹配参数 ", "测试效果"}."测试效果" ("Main")) -> ()  [unwired: 2 in, 2 out]
        n104 = call "Enqueue Element Array.vi"("priority"=w294, "queue index"=0, "error in"=w291, "master data"="测试按钮", "queue in"=w292) -> ("error out"=w289:errorcluster, "queue out"=w290:T8)  [unwired: 5 in]
      }
      event "刷新": Value Change {
        n105 = event-data() -> ()  [unwired: 1 in, 6 out]
        n106 = disable-structure shown="禁用" {
          disable-tunnel: w300 -> [w304 _]
          disable-tunnel: w299 -> [w303 _]
          disable-tunnel: [w302 _] -> w298
          disable-tunnel: [w301 _] -> w297
          frame Disabled {
            w306 = u16 1 items=["HPRI"=1, "LPRI"=0] ("priority")
            # "刷新"
            n107 = call "Enqueue Element Array.vi"("priority"=w306, "queue index"=0, "error in"=w303, "master data"="刷新", "queue in"=w304) -> ("error out"=w301:errorcluster, "queue out"=w302:T8)  [unwired: 5 in]
          }
          frame Enabled {
          }
        }
        n108 = property on="Main" class="TabCtl (严格)"("Value"=enum32{"主参数", "模板匹配参数 ", "测试效果"}."模板匹配参数 " ("Main")) -> ()  [unwired: 2 in, 2 out]
      }
    }
    n109 = call "GetSystemTime.vi"() -> ("date/time string"=→"system time":string)  [unwired: 7 in]
  }
  n110 = call "Release Queue Array.vi"("error in"=w3, "queue in"=w1) -> ("error out"=w2:errorcluster)  [unwired: 2 in, 3 out]
  n111 = call "Release Queue Array.vi"("error in"=w6, "queue in"=w1) -> ("error out"=w9:errorcluster)  [unwired: 2 in, 3 out]
  n112 = call "MergeErrors.vi"("error in 3 (no error)"=w2, "error in 4 (no error)"=w9) -> ("error out"=w8:errorcluster)  [unwired: 6 in]
  n113 = call "ExitAppMode.vi"("error in (no error)"=w8) -> ("error out"=w7:errorcluster)  [unwired: 10 in]
  n114 = call <vilib>:"Clear Errors.vi"("error in (no error)"=w7) -> ()  [unwired: 5 in, 2 out]
